vi "603xA Set Mask Register.vi"(0 "VISA resource name":refnum<visa-resource-name>, 1 "ac line dropout (F:off)":bool, 2 "overtemperature (F:off)":bool, 3 "overvoltage (F:off)":bool, 5 "remote inhibit (F:off)":bool, 7 "error (F:off)":bool, 9 "foldback (F:off)":bool, 11 "error in (no error)":errorcluster, 12 "overrange (F:off)":bool, 13 "cc mode (F:off)":bool, 14 "cv mode (F:off)":bool) -> (4 "VISA resource name out":refnum<visa-resource-name>, 15 "error out":errorcluster)   [LabVIEW 2020, in "Agilent 6XXX Series.lvlib"]
doc: "This function sets the mask register which specifies which bits in the status register are enabled to set bits in the fault register. Basically, this function allows the operator to define which conditions are fault conditions."
uses:
  <instrlib>/Agilent 6XXX Series/Agilent 6XXX Series.lvlib
panel:
  # "HP603XA series only"
  # "Set Mask for.."
  # "on\noff"
  # "on\noff"
  # "on\noff"
  # "on\noff"
  # "on\noff"
  # "on\noff"
  # "on\noff"
  # "on\noff"
  # "on\noff"
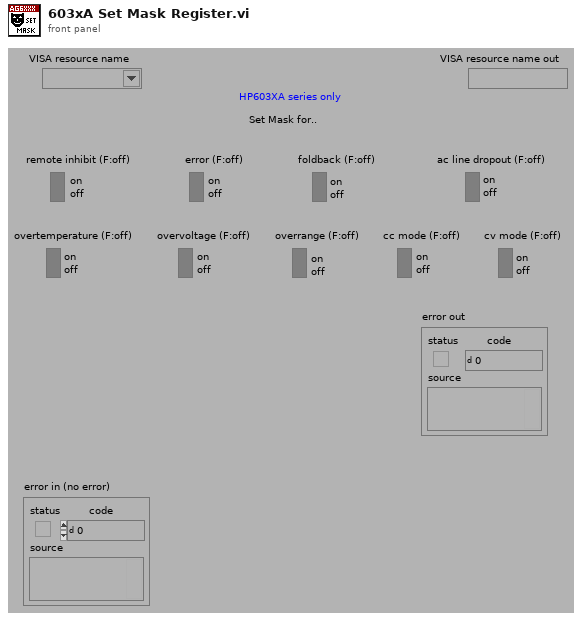
[diagram p1: front panel]
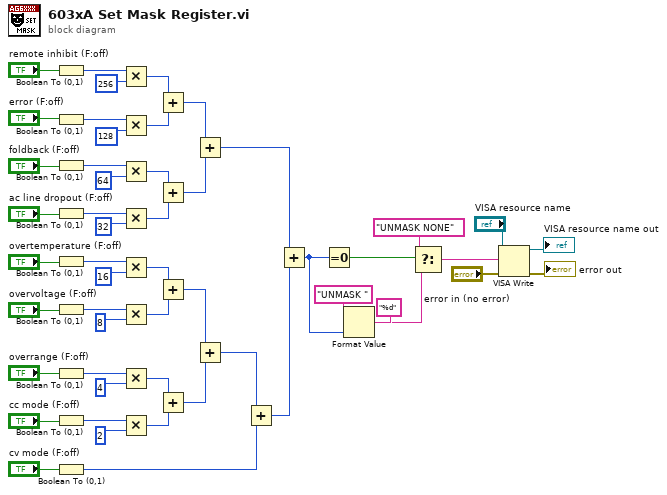
[diagram p0: block diagram]
diagram:
  n1 = Boolean To (0,1)(Boolean="remote inhibit (F:off)") -> (0, 1=w43:i16)
  n2 = Boolean To (0,1)(Boolean="error (F:off)") -> (0, 1=w42:i16)
  n3 = Boolean To (0,1)(Boolean="foldback (F:off)") -> (0, 1=w41:i16)
  n4 = Boolean To (0,1)(Boolean="ac line dropout (F:off)") -> (0, 1=w40:i16)
  n5 = Boolean To (0,1)(Boolean="overtemperature (F:off)") -> (0, 1=w39:i16)
  n6 = Boolean To (0,1)(Boolean="overvoltage (F:off)") -> (0, 1=w38:i16)
  n7 = Boolean To (0,1)(Boolean="overrange (F:off)") -> (0, 1=w37:i16)
  n8 = Boolean To (0,1)(Boolean="cc mode (F:off)") -> (0, 1=w36:i16)
  n9 = Boolean To (0,1)(Boolean="cv mode (F:off)") -> (0, 1=w15:i16)
  n10 = Multiply(x=w43, y=i16 256) -> (x*y=w27:i16)
  n11 = Multiply(x=w42, y=i16 128) -> (x*y=w26:i16)
  n12 = Multiply(x=w41, y=i16 64) -> (x*y=w25:i16)
  n13 = Multiply(x=w40, y=i16 32) -> (x*y=w24:i16)
  n14 = Multiply(x=w39, y=i16 16) -> (x*y=w23:i16)
  n15 = Multiply(x=w38, y=i16 8) -> (x*y=w22:i16)
  n16 = Multiply(x=w37, y=i16 4) -> (x*y=w21:i16)
  n17 = Multiply(x=w36, y=i16 2) -> (x*y=w20:i16)
  n18 = Add(x=w27, y=w26) -> (x+y=w16:i16)
  n19 = Add(x=w25, y=w24) -> (x+y=w17:i16)
  n20 = Add(x=w23, y=w22) -> (x+y=w18:i16)
  n21 = Add(x=w21, y=w20) -> (x+y=w19:i16)
  n22 = Add(x=w16, y=w17) -> (x+y=w13:i16)
  n23 = Add(x=w18, y=w19) -> (x+y=w14:i16)
  n24 = Add(x=w14, y=w15) -> (x+y=w12:i16)
  n25 = Add(x=w13, y=w12) -> (x+y=w9:i16)
  n26 = Equal To 0?(x=w9) -> (x = 0?=w11:bool)
  n27 = Format Value(string ("")="UNMASK ", format string="%d", value (0)=w9) -> (output string=w6:string)
  n28 = Select(t="UNMASK NONE", s=w11, f=w6) -> (s? t:f=w5:string)
  n29 = VISA Write(VISA resource name="VISA resource name", write buffer=w5, error in (no error)="error in (no error)") -> (VISA resource name out=→"VISA resource name out":refnum<visa-resource-name>, error out=→"error out":errorcluster)  [unwired: 1 out]
